vi "Convert Binary file to Text.vi"(7 "Originating directory":path, 8 "error in (no error)":errorcluster, 10 "TDMS File Path":path, 11 "Destination directory":path) -> (0 "error out":errorcluster)   [LabVIEW 2010, in "TDMS to ASCII Convert.lvlib"]
uses:
  TDMS to ASCII Convert.lvlib
  Open NIVS TDMS log.vi
  Calculate Current Read Size.vi
  Create Ascii Header.vi
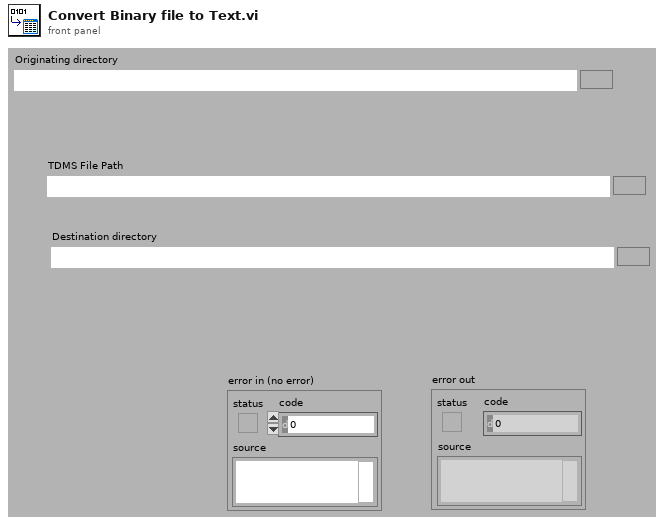
[diagram p1: front panel]
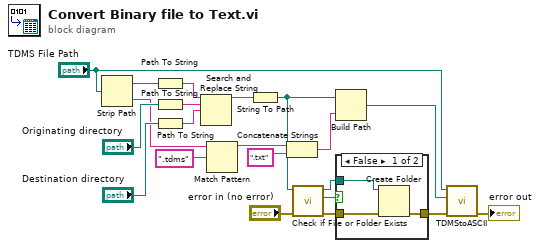
[diagram p0: block diagram]
diagram:
  n1 = Strip Path(path="TDMS File Path") -> (stripped path=w6:path, name=w8:string)
  n2 = Path To String(path=w6) -> (string=w17:string)
  n3 = Path To String(path="Originating directory") -> (string=w16:string)
  n4 = Path To String(path="Destination directory") -> (string=w15:string)
  n5 = Search and Replace String(input string=w17, search string=w16, replace string=w15) -> (result string=w14:string)  [unwired: 5 in, 3 out]
  n6 = Match Pattern(string=w8, regular expression=".tdms") -> (before substring=w7:string)  [unwired: 1 in, 3 out]
  n7 = String To Path(string=w14) -> (path=w13:path)
  n8 = Concatenate Strings(w7, ".txt" ("string")) -> (w20:string)
  n9 = call <vilib>:"Check if File or Folder Exists.vi"("error in (no error)"="error in (no error)", "path"=w13) -> ("error out"=w11:errorcluster, "file or folder exists?"=w10:bool, "dup path"=w12:path)  [unwired: 7 in]
  n10 = Build Path(base path=w13, name or relative path=w20) -> (appended path=w5:path)
  n11 = case shown="False" w10 {
    tunnel: [w24 w25] -> w2
    tunnel: w12 -> [w23 _]
    tunnel: w11 -> [w22 w25]
    frame False {
      n12 = Create Folder(path (use dialog)=w23, error in=w22) -> (error out=w24:errorcluster)  [unwired: 1 in, 2 out]
    }
    frame True {
    }
  }
  n13 = call "TDMStoASCII.vi"("error in (no error)"=w2, "Ascii file to write"=w5, "TDMS File"="TDMS File Path") -> ("error out"=→"error out":errorcluster)  [unwired: 8 in]
